vi "ERIO RT Check State Change.vi"(9 "RT Current State In":T1, 10 "RT Previous State":T1) -> (1 "RT Current State Out":T1, 2 "Alarm-Notifier Action":T4=enum."Into Shutdown")   [LabVIEW 2017]
doc: "Checks for a state change and provides related indications from results. \n\nJames Tillett P.E.\nEndeavor Engineering Inc.\nwww.endeavoreng.com"
uses:
  Controls/ERIO RT State Variables.ctl
  Controls/ERIO SystemStates.ctl
  Controls/ERIO Queue Data.ctl
  Controls/ERIO Worker Variables.ctl
  Controls/ERIO Alarm-Notifier Action.ctl
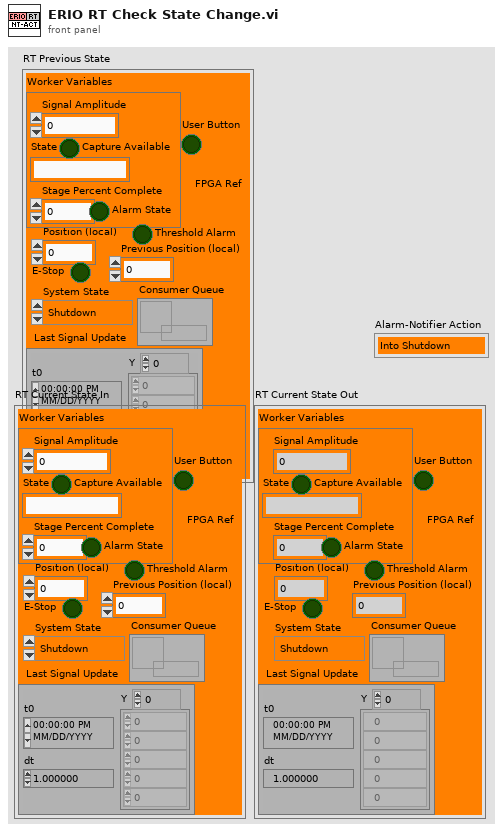
[diagram p1: front panel]
types:
  T1 = typedef "ERIO RT State Variables.ctl" = cluster{"Position (local)":i16, "E-Stop":bool, "System State":T2, "FPGA Ref":refnum<k20>, "Previous Position (local)":i16, "Consumer Queue":refnum<queue>, "Worker Variables":T3, "Threshold Alarm":bool, "User Button":bool, "Last Signal Update":waveform(dbl)}
  T2 = typedef "ERIO SystemStates.ctl" = enum16{"Shutdown", "E-STOP", "Reset Process", "Stage 1", "Stage 2", "Stage 3", "Alarm State"}
  T3 = typedef "ERIO Worker Variables.ctl" = cluster{"Signal Amplitude":dbl, "State":string, "Stage Percent Complete":dbl, "Alarm State":bool, "Capture Available":bool}
  T4 = typedef "ERIO Alarm-Notifier Action.ctl" = enum16{"No Action", "Threshold Alarm", "Into Stage 1", "Into Stage 2", "Into Stage 3", "Into Shutdown", "Into Process Reset", "Into E-STOP", "User Button"}
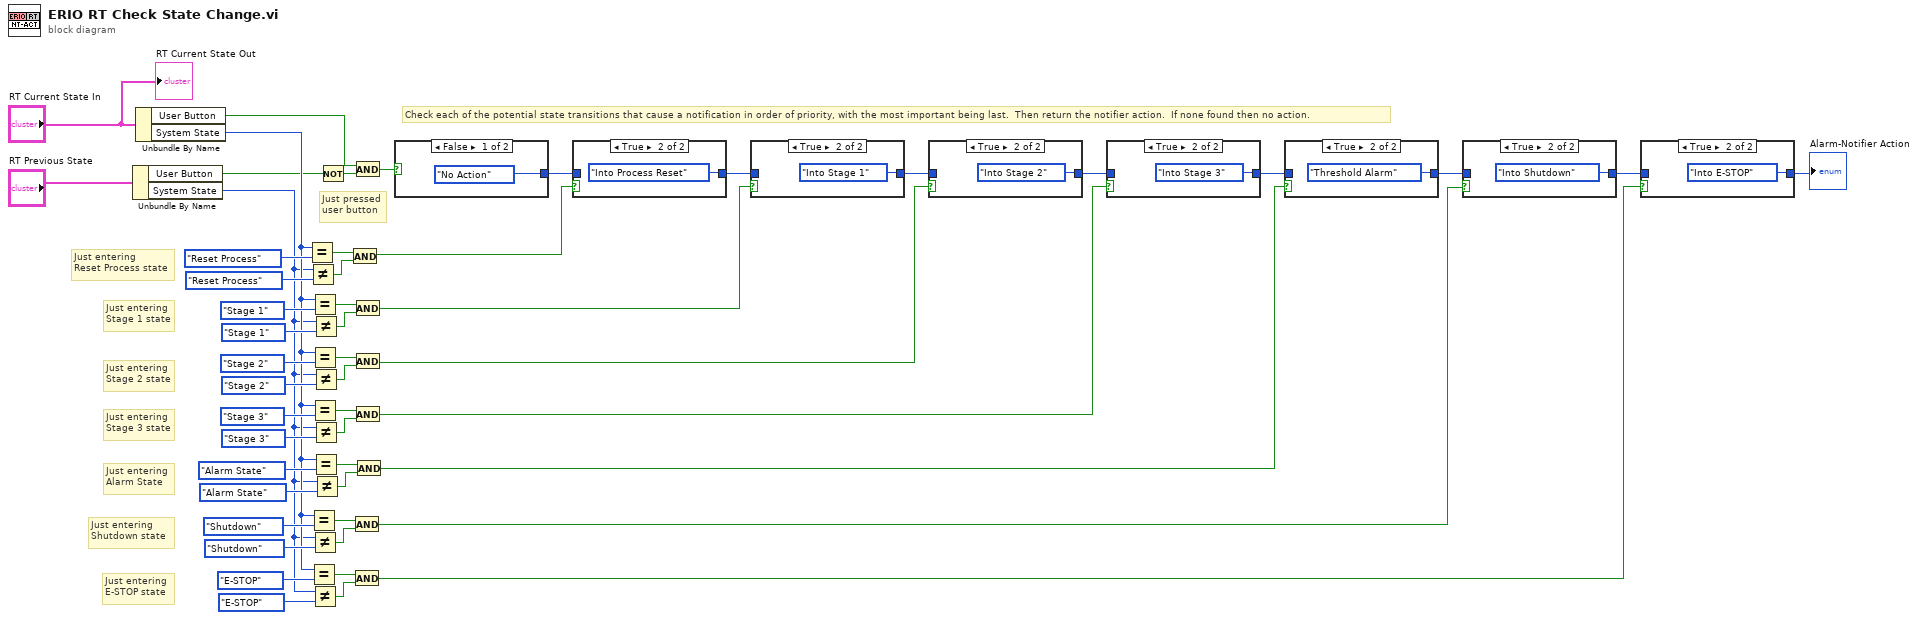
[diagram p0: block diagram]
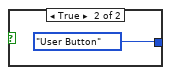
[diagram p9: hidden frame]
diagram:
  # "Check each of the potential state transitions that cause a notification in order of priority, with the most important being last.  Then return the notifier action.  If none found then no action."
  # "Just pressed\nuser button"
  # "Just entering\nAlarm State"
  # "Just entering\nE-STOP state"
  # "Just entering\nShutdown state"
  # "Just entering\nStage 3 state"
  # "Just entering\nStage 2 state"
  # "Just entering\nStage 1 state"
  # "Just entering\nReset Process state"
  n1 = Unbundle By Name("RT Previous State") -> ("User Button"=w20:bool, "System State"=w21:T2)
  n2 = Unbundle By Name("RT Current State In") -> ("User Button"=w18:bool, "System State"=w22:T2)
  n3 = Equal?(x=w22, y=ERIO_SystemStates."Reset Process" ("System State")) -> (x = y?=w48:bool)
  n4 = Not Equal?(x=w21, y=ERIO_SystemStates."Reset Process" ("System State")) -> (x != y?=w47:bool)
  n5 = Equal?(x=w22, y=ERIO_SystemStates."Shutdown" ("System State")) -> (x = y?=w28:bool)
  n6 = Equal?(x=w22, y=ERIO_SystemStates."E-STOP" ("System State")) -> (x = y?=w29:bool)
  n7 = Equal?(x=w22, y=ERIO_SystemStates."Stage 1" ("System State")) -> (x = y?=w45:bool)
  n8 = Equal?(x=w22, y=ERIO_SystemStates."Stage 2" ("System State")) -> (x = y?=w40:bool)
  n9 = Equal?(x=w22, y=ERIO_SystemStates."Stage 3" ("System State")) -> (x = y?=w27:bool)
  n10 = Not Equal?(x=w21, y=ERIO_SystemStates."Shutdown" ("System State")) -> (x != y?=w33:bool)
  n11 = Not Equal?(x=w21, y=ERIO_SystemStates."E-STOP" ("System State")) -> (x != y?=w32:bool)
  n12 = Not Equal?(x=w21, y=ERIO_SystemStates."Stage 1" ("System State")) -> (x != y?=w46:bool)
  n13 = Not Equal?(x=w21, y=ERIO_SystemStates."Stage 2" ("System State")) -> (x != y?=w39:bool)
  n14 = Not Equal?(x=w21, y=ERIO_SystemStates."Stage 3" ("System State")) -> (x != y?=w38:bool)
  n15 = Equal?(x=w22, y=ERIO_SystemStates."Alarm State" ("System State")) -> (x = y?=w26:bool)
  n16 = Not Equal?(x=w21, y=ERIO_SystemStates."Alarm State" ("System State")) -> (x != y?=w23:bool)
  n17 = Not(x=w20) -> (.not. x?=w19:bool)
  n18 = And(x=w48, y=w47) -> (x .and. y?=w9:bool)
  n19 = And(x=w28, y=w33) -> (x .and. y?=w4:bool)
  n20 = And(x=w29, y=w32) -> (x .and. y?=w3:bool)
  n21 = And(x=w18, y=w19) -> (x .and. y?=w10:bool)
  n22 = And(x=w45, y=w46) -> (x .and. y?=w8:bool)
  n23 = And(x=w40, y=w39) -> (x .and. y?=w7:bool)
  n24 = And(x=w27, y=w38) -> (x .and. y?=w6:bool)
  n25 = And(x=w26, y=w23) -> (x .and. y?=w5:bool)
  n26 = case shown="False" w10 {
    tunnel: [ERIO_Alarm-Notifier_Action."No Action" ("Alarm-Notifier Action") ERIO_Alarm-Notifier_Action."User Button" ("Alarm-Notifier Action")] -> w17
    frame False {
    }
    frame True {
    }
  }
  n27 = case shown="True" w9 {
    tunnel: [w54 ERIO_Alarm-Notifier_Action."Into Process Reset" ("Alarm-Notifier Action")] -> w16
    tunnel: w17 -> [w54 _]
    frame False {
    }
    frame True {
    }
  }
  n28 = case shown="True" w8 {
    tunnel: [w56 ERIO_Alarm-Notifier_Action."Into Stage 1" ("Alarm-Notifier Action")] -> w15
    tunnel: w16 -> [w56 _]
    frame False {
    }
    frame True {
    }
  }
  n29 = case shown="True" w7 {
    tunnel: [w58 ERIO_Alarm-Notifier_Action."Into Stage 2" ("Alarm-Notifier Action")] -> w14
    tunnel: w15 -> [w58 _]
    frame False {
    }
    frame True {
    }
  }
  n30 = case shown="True" w6 {
    tunnel: [w60 ERIO_Alarm-Notifier_Action."Into Stage 3" ("Alarm-Notifier Action")] -> w13
    tunnel: w14 -> [w60 _]
    frame False {
    }
    frame True {
    }
  }
  n31 = case shown="True" w5 {
    tunnel: [w62 ERIO_Alarm-Notifier_Action."Threshold Alarm" ("Alarm-Notifier Action")] -> w12
    tunnel: w13 -> [w62 _]
    frame False {
    }
    frame True {
    }
  }
  n32 = case shown="True" w4 {
    tunnel: [w64 ERIO_Alarm-Notifier_Action."Into Shutdown" ("Alarm-Notifier Action")] -> w11
    tunnel: w12 -> [w64 _]
    frame False {
    }
    frame True {
    }
  }
  n33 = case shown="True" w3 {
    tunnel: [w66 ERIO_Alarm-Notifier_Action."Into E-STOP" ("Alarm-Notifier Action")] -> w2
    tunnel: w11 -> [w66 _]
    frame False {
    }
    frame True {
    }
  }
  "Alarm-Notifier Action" <- w2
  "RT Current State Out" <- "RT Current State In"
